vi "Connect.vi"(11 "Connection ID":T1) -> (2 "Connect?":bool, 3 "Connection ID Out":T1)   [LabVIEW 2017, in "GL860_Driver.lvlib"]
uses:
  GL860_Driver.lvlib
  Driver/ConnectionID.ctl
  Driver/GLdrv_Open_USB.vi
  Driver/GLdrv_Open_TCPIP.vi
panel:
  in  "閉じる":bool
  in  "切断":bool
  in  "接続":bool
  in  "SEL":enum32{"USB", "LAN"}(tab)
  in  "USB ID":i32 min=0 max=31
  in  "IPアドレス まはた ドメイン":string="192.168.0.100"
  in  "ポート":u16=8023
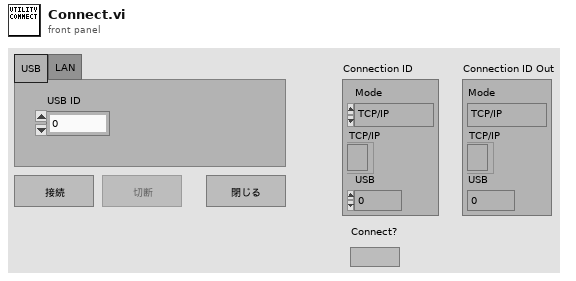
[diagram p1: front panel]
types:
  T1 = typedef "ConnectionID.ctl" = cluster{"Mode":enum16{"TCP/IP", "USB"}, "TCP/IP":refnum<k5>, "USB":i32}
  T2 = enum8{"Enabled", "Disabled", "Disabled and Grayed Out"}
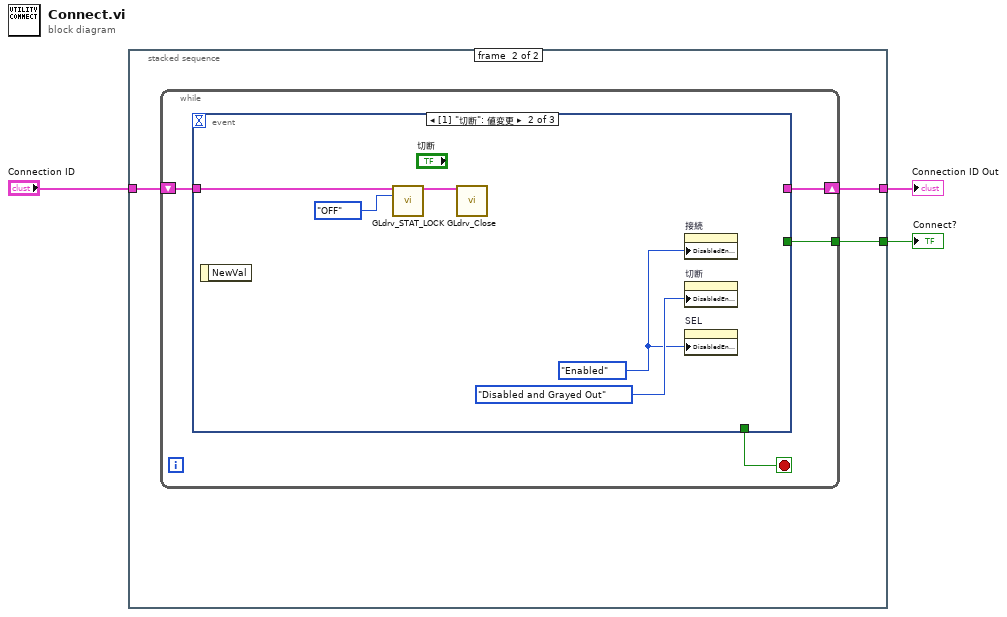
[diagram p0: block diagram]
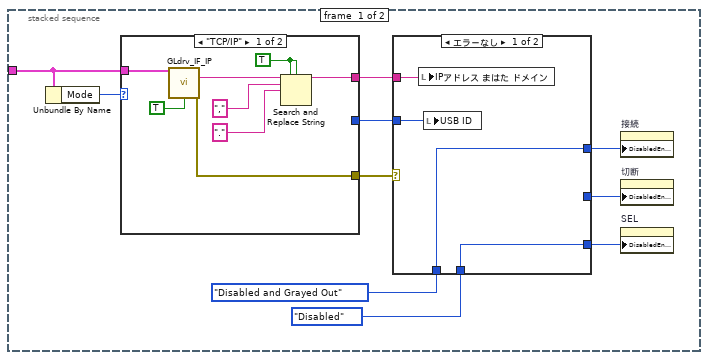
[diagram p2: hidden frame]
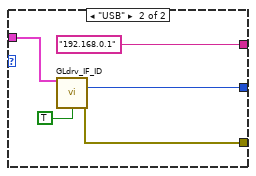
[diagram p4: hidden frame]
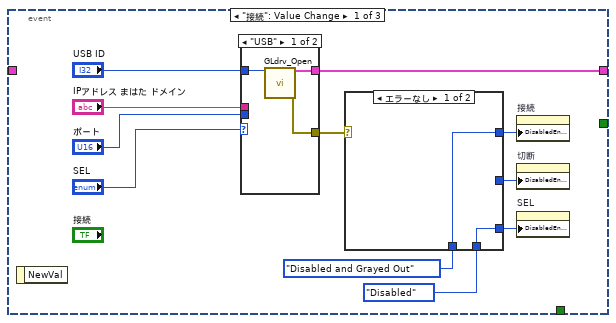
[diagram p5: hidden frame]
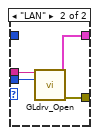
[diagram p6: hidden frame]
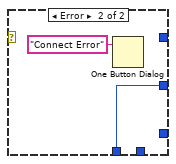
[diagram p7: hidden frame]
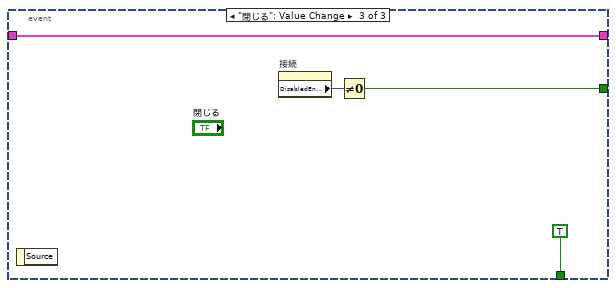
[diagram p8: hidden frame]
diagram:
  n1 = stacked-sequence {
    tunnel: "Connection ID" -> [w13 w34]
    tunnel: [_ w33] -> w2
    tunnel: [_ w32] -> w1
    frame #0 {
      n2 = Unbundle By Name(w13) -> ("Mode"=w12:enum16{"TCP/IP", "USB"})
      n3 = case shown="\"TCP/IP\"" w12 {
        tunnel: w13 -> [w26 w30]
        tunnel: [w22 "192.168.0.1" ("IP out")] -> w4
        tunnel: [_ w29] -> w5
        tunnel: [w25 w28] -> w11
        frame "TCP/IP" {
          w19 = TRUE ("replace all? (F)")
          n4 = call "GLdrv_IF_IP.vi"("Connection ID"=w26, "Query(f)"=TRUE) -> ("IP out"=w23:string, "error out"=w25:errorcluster)  [unwired: 11 in, 1 out]
          n5 = Search and Replace String(replace all?=w19, case sensitive?=w19, input string=w23, search string=",", replace string="." ("search string")) -> (result string=w22:string)  [unwired: 3 in, 3 out]
        }
        frame "USB" {
          n6 = call "GLdrv_IF_ID.vi"("Connection ID"=w30, "Query(f)"=TRUE) -> ("ID out"=w29:i32, "error out"=w28:errorcluster)  [unwired: 11 in, 1 out]
        }
      }
      n7 = case shown="エラーなし" w11 {
        tunnel: T2."Disabled and Grayed Out" ("Disabled") -> [w17 w18]
        tunnel: [_ w18] -> w9
        tunnel: [w17 _] -> w8
        tunnel: [w16 _] -> w7
        tunnel: T2."Disabled" ("Disabled") -> [w16 _]
        tunnel: w5 -> [w15 _]
        tunnel: w4 -> [w14 _]
        frame No Error {
          n8 = local write "IPアドレス まはた ドメイン"(w14) -> ()
          n9 = local write "USB ID"(w15) -> ()
        }
        frame Error {
        }
      }
      n10 = property on="接続" class="Bool"("DisabledEnum"=w8) -> ()  [unwired: 2 in, 2 out]
      n11 = property on="切断" class="Bool"("DisabledEnum"=w9) -> ()  [unwired: 2 in, 2 out]
      n12 = property on="SEL" class="TabCtl （指定）"("DisabledEnum"=w7) -> ()  [unwired: 2 in, 2 out]
    }
    frame #1 {
      n13 = while {
        shift-right: [w37] -> w33
        shift-left: w34 -> [w36]
        tunnel: [w35] -> w32
        stop <- w38 stop-if-true
        n14 = event shown="[1] \"切断\": 値変更" {
          selector: _ -> [_ _ _]
          dyn-events: _ -> [_ _ _]
          timeout: _ -> [_ _ _]
          tunnel: [_ _ TRUE] -> w38
          tunnel: [w45 _ w68] -> w37
          tunnel: w36 -> [_ w62 w68]
          tunnel: [_ _ w66] -> w35
          event "接続": Value Change {
            n15 = event-data() -> ()  [unwired: 1 in, 1 out]
            n16 = case shown="\"USB\"" "SEL" {
              tunnel: [w52 w56] -> w45
              tunnel: [w51 w55] -> w44
              tunnel: "USB ID" -> [w50 _]
              tunnel: "IPアドレス まはた ドメイン" -> [_ w54]
              tunnel: "ポート" -> [_ w53]
              frame "USB" {
                n17 = call-poly "GLdrv_Open.vi"("ID"=w50) -> ("Connection ID"=w52:T1, "error out"=w51:errorcluster)  [unwired: 13 in]
              }
              frame "LAN" {
                n18 = call-poly "GLdrv_Open.vi"("address"=w54, "remote port"=w53) -> ("Connection ID"=w56:T1, "error out"=w55:errorcluster)  [unwired: 12 in]
              }
            }
            n19 = case shown="エラーなし" w44 {
              tunnel: T2."Disabled and Grayed Out" ("Disabled") -> [w58 w60]
              tunnel: [w58 _] -> w48
              tunnel: [_ w60] -> w47
              tunnel: [w57 _] -> w46
              tunnel: T2."Disabled" ("Disabled") -> [w57 _]
              frame No Error {
              }
              frame Error {
                n20 = One Button Dialog(message="Connect Error") -> ()  [unwired: 1 in, 1 out]
              }
            }
            n21 = property on="接続" class="Bool"("DisabledEnum"=w48) -> ()  [unwired: 2 in, 2 out]
            n22 = property on="切断" class="Bool"("DisabledEnum"=w47) -> ()  [unwired: 2 in, 2 out]
            n23 = property on="SEL" class="TabCtl （指定）"("DisabledEnum"=w46) -> ()  [unwired: 2 in, 2 out]
          }
          event "切断": Value Change {
            w64 = T2."Enabled" ("Disabled")
            n24 = event-data() -> ()  [unwired: 1 in, 1 out]
            n25 = call "GLdrv_STAT_LOCK.vi"("Connection ID"=w62, "LOCK"=enum16{"ON", "OFF"}."OFF") -> ("Connection ID Out"=w63:T1)  [unwired: 11 in, 2 out]
            n26 = call "GLdrv_Close.vi"("Connection ID Out"=w63) -> ()  [unwired: 14 in, 1 out]
            n27 = property on="接続" class="Bool"("DisabledEnum"=w64) -> ()  [unwired: 2 in, 2 out]
            n28 = property on="切断" class="Bool"("DisabledEnum"=T2."Disabled and Grayed Out" ("Disabled")) -> ()  [unwired: 2 in, 2 out]
            n29 = property on="SEL" class="TabCtl （指定）"("DisabledEnum"=w64) -> ()  [unwired: 2 in, 2 out]
          }
          event "閉じる": Value Change {
            n30 = event-data() -> ()  [unwired: 1 in, 1 out]
            n31 = property on="接続" class="Bool"() -> ("DisabledEnum"=w67:T2)  [unwired: 2 in, 2 out]
            n32 = Not Equal To 0?(x=w67) -> (x != 0?=w66:bool)
          }
        }
      }
    }
  }
  "Connection ID Out" <- w2
  "Connect?" <- w1
